vi "Get semaphore.vi"(11 "arm in":refnum<class "arm.lvclass">) -> (2 "semaphore":T1, 3 "arm out":refnum<class "arm.lvclass">)   [LabVIEW 2015, in "arm.lvclass"]
uses:
  arm.lvclass
  arm.lvclass/arm.ctl
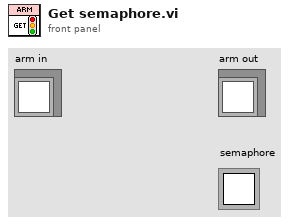
[diagram p1: front panel]
types:
  T1 = typedef "Semaphore RefNum" = refnum<k1>
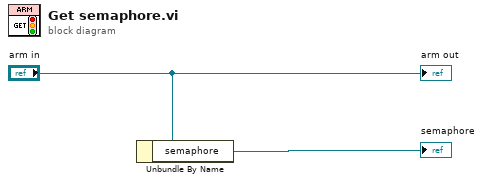
[diagram p0: block diagram]
diagram:
  n1 = Unbundle By Name("arm in") -> ("semaphore"=→"semaphore":T1)
  "arm out" <- "arm in"
